vi "GetVoltageBuseProperties.vi"(8 "error in (no error)":errorcluster, 10 "Channel Properties":T2[](array[typedef])) -> (0 "error out":errorcluster, 3 "VoltageBus":T1)   [LabVIEW 2017, in "McsaVirtualChannel.lvlib"]
uses:
  <vilib>/addons/InsightCM/Devices/Shared/Mcsa/McsaVirtualChannel/McsaVirtualChannel.lvlib
  <vilib>/addons/InsightCM/MessageBus/Base/controls/KeyValuePair.ctl
  <vilib>/addons/InsightCM/Devices/Shared/Mcsa/McsaVirtualChannel/controls/VoltageBus.ctl
  <vilib>/addons/InsightCM/Utilities/PropertyHelpers/PropertyHelpers.lvlib
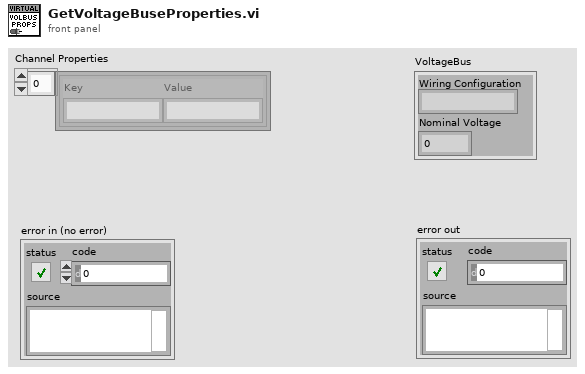
[diagram p1: front panel]
types:
  T1 = typedef "McsaVirtualChannel.lvlib/VoltageBus.ctl" = cluster{"Wiring Configuration":string, "Nominal Voltage":dbl}
  T2 = typedef "KeyValuePair.ctl" = cluster{"Key":string, "Value":string}
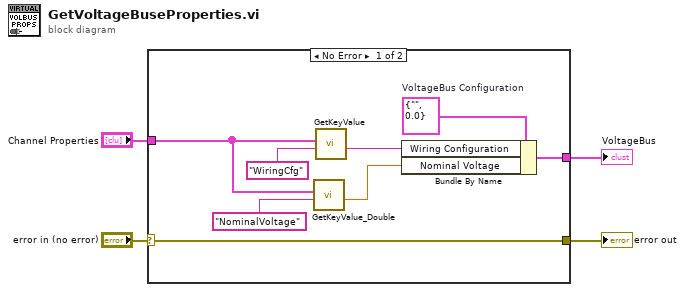
[diagram p0: block diagram]
diagram:
  n1 = case shown="No Error" "error in (no error)" {
    selector: "error in (no error)" -> [w8 _]
    tunnel: "Channel Properties" -> [w6 _]
    tunnel: [w10 _] -> w3
    tunnel: [w8 _] -> w1
    frame No Error {
      w11 = T1 {"Wiring Configuration"="", "Nominal Voltage"=0.0}  # VoltageBus Configuration
      n2 = call <vilib>:"GetKeyValue_Double.vi"("key"="NominalVoltage" ("name"), "key value pairs"=w6) -> ("value"=w5:dbl)  [unwired: 7 in, 2 out]
      n3 = call <vilib>:"GetKeyValue.vi"("key"="WiringCfg" ("name"), "key value pairs"=w6) -> ("value"=w9:string)  [unwired: 7 in, 2 out]
      n4 = Bundle By Name(cluster=w11, "Wiring Configuration"=w9, "Nominal Voltage"=w5) -> (w10:T1)
    }
    frame Error {
    }
  }
  "error out" <- w1
  "VoltageBus" <- w3
